vi "File.Get App List.vi"(10 "Type":enum16{"32 Bit", "64 Bit"}(ring), 11 "Prg Folder":string="Valve") -> (2 "App List":T1[](array[typedef]), 3 "Available Applications":string[](array[string]))   [LabVIEW 2018]
uses:
  File.Name and Path List Itemctl.ctl
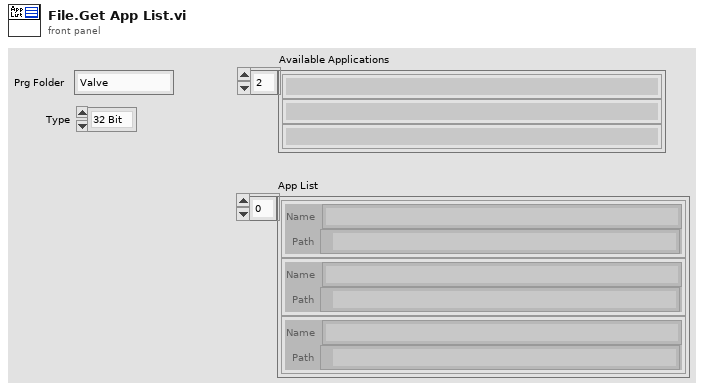
[diagram p1: front panel]
types:
  T1 = typedef "File.Name and Path List Itemctl.ctl" = cluster{"Name":string, "Path":path}
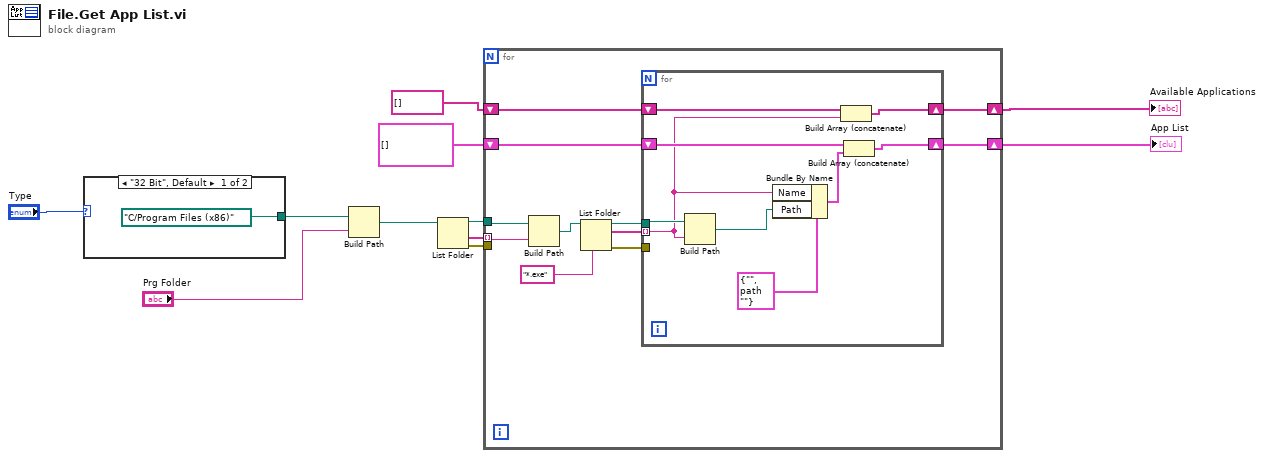
[diagram p0: block diagram]
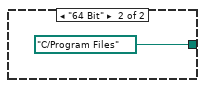
[diagram p2: hidden frame]
diagram:
  n1 = case shown="\"32 Bit\", Default" "Type" {
    tunnel: [path "C:/Program Files (x86)" path "C:/Program Files"] -> w10
    frame "32 Bit", Default {
    }
    frame "64 Bit" {
    }
  }
  n2 = Build Path(base path=w10, name or relative path="Prg Folder") -> (appended path=w8:path)
  n3 = List Folder(path=w8) -> (path out=w7:path, folder names=w6:string[], error out=w5:errorcluster)  [unwired: 3 in, 1 out]
  n4 = for {
    tunnel: w7 -> [w23]
    tunnel: w6 -> [w22] mode=indexing
    tunnel: w5 -> [_]
    shift-right: [w16] -> w3
    shift-left: T1[] [] ("App List") -> [w17]
    shift-right: [w15] -> w1
    shift-left: string[] [] ("Available Applications") -> [w14]
    n5 = Build Path(base path=w23, name or relative path=w22) -> (appended path=w21:path)
    n6 = List Folder(path=w21, pattern="*.exe") -> (path out=w19:path, filenames=w20:string[], error out=w18:errorcluster)  [unwired: 2 in, 1 out]
    n7 = for {
      tunnel: w20 -> [w25] mode=indexing
      tunnel: w19 -> [w33]
      tunnel: w18 -> [_]
      shift-right: [w28] -> w16
      shift-left: w17 -> [w32]
      shift-right: [w27] -> w15
      shift-left: w14 -> [w26]
      n8 = Build Path(base path=w33, name or relative path=w25) -> (appended path=w30:path)
      n9 = Bundle By Name(cluster=T1 {"Name"="", "Path"=path ""} ("App"), "Name"=w25, "Path"=w30) -> (w29:T1)
      n10 = Build Array (concatenate)(w26, w25) -> (w27:string[])
      n11 = Build Array (concatenate)(w32, w29) -> (w28:T1[])
    }
  }
  "Available Applications" <- w1
  "App List" <- w3
